vi "NI USB GPIB Command.vi"(4 "Error In":errorcluster, 5 "Wait for instrument to respond (s)":dbl, 6 "String to Send":string="C0", 7 "VISA resource name":refnum<visa-resource-name>="GPIB1::25::INSTR") -> (0 "Error Out":errorcluster={"status"=TRUE, "code"=-1073807339, "source"="VISA Read in NI USB GPIB Command.vi"}, 1 "Return String from Device (Not all commands return a String)":string="C\r", 2 "Number of Bytes Recieved at Serial Port":u32, 3 "VISA resource name out":refnum<visa-resource-name>)   [LabVIEW 2016, in "IPS-120.lvlib"]
uses:
  IPS-120.lvlib
panel:
  out "return count":u32
  out "Number of Bytes sent":u32=4
  # "NI Example Serial Code"
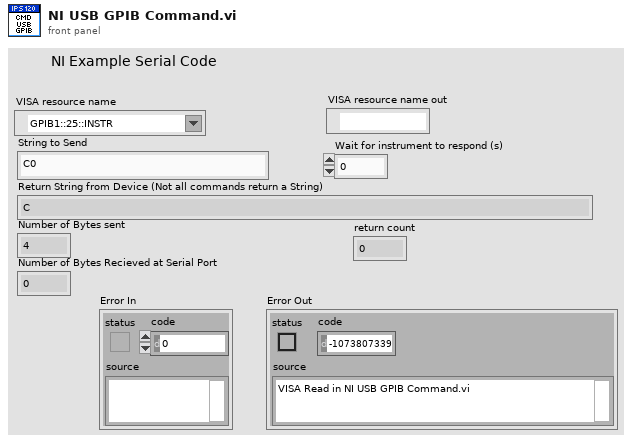
[diagram p1: front panel]
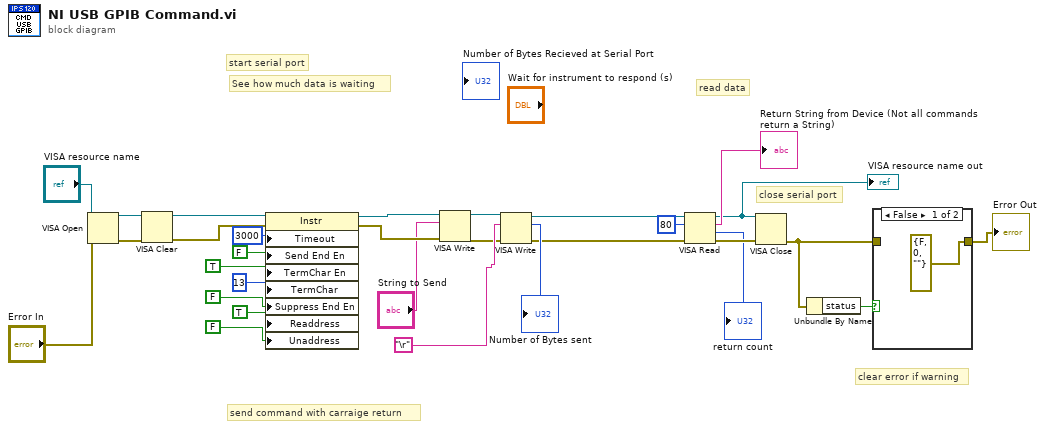
[diagram p0: block diagram]
diagram:
  # "clear error if warning"
  # "close serial port"
  # "read data"
  # "See how much data is waiting"
  # "send command with carraige return"
  # "start serial port"
  n1 = VISA Open(error in (no error)="Error In", VISA resource name="VISA resource name") -> (VISA resource name=w18:refnum<visa-resource-name>, error out=w19:errorcluster)  [unwired: 3 in]
  n2 = VISA Clear(VISA resource name=w18, error in (no error)=w19) -> (VISA resource name out=w16:refnum<visa-resource-name>, error out=w17:errorcluster)
  n3 = property class="Instr"(reference=w16, error in=w17, "Timeout"=u32 3000 ("General Settings:Timeout Value"), "Send End En"=FALSE ("Message Based Settings:Send End Enable"), "TermChar En"=TRUE ("Message Based Settings:Termination Character Enable"), "TermChar"=u8 13 ("Message Based Settings:Termination Character"), "Suppress End En"=FALSE ("Message Based Settings:Suppress End Enable"), "Readdress"=TRUE ("GPIB Settings:Readdressing"), "Unaddress"=FALSE ("GPIB Settings:Unaddressing")) -> (reference out=w14:refnum<visa-resource-name>, error out=w15:errorcluster)
  n4 = VISA Write(VISA resource name=w14, write buffer="String to Send", error in (no error)=w15) -> (VISA resource name out=w10:refnum<visa-resource-name>, error out=w11:errorcluster)  [unwired: 1 out]
  n5 = VISA Write(VISA resource name=w10, write buffer="\r", error in (no error)=w11) -> (VISA resource name out=w28:refnum<visa-resource-name>, return count=→"Number of Bytes sent":u32, error out=w26:errorcluster)
  n6 = VISA Read(VISA resource name=w28, byte count=u32 80, error in (no error)=w26) -> (VISA resource name out=w6:refnum<visa-resource-name>, read buffer=→"Return String from Device (Not all commands return a String)":string, return count=→"return count":u32, error out=w30:errorcluster)
  "VISA resource name out" <- w6
  n7 = VISA Close(VISA resource name=w6, error in (no error)=w30) -> (error out=w1:errorcluster)
  n8 = Unbundle By Name(w1) -> ("status"=w3:bool)
  n9 = case shown="False" w3 {
    tunnel: [errorcluster {"status"=FALSE, "code"=0, "source"=""} ("error constant") w32] -> w2
    tunnel: w1 -> [_ w32]
    frame False {
    }
    frame True {
    }
  }
  "Error Out" <- w2
